vi "newOdometry.vi"(8 "Wheel angles":dbl[](array[numeric]), 9 "Wheel speed":dbl[](array[numeric]), 10 "prevSTR":dbl, 11 "prevFWD":dbl) -> (1 "Strafe":dbl, 2 "Forward":dbl)   [LabVIEW 2020]
uses:
  <vilib>/Rock Robotics/WPI/ThirdParty/Sensors/navX/_TypeDefs/FRIC_navX_DeviceNumbersTypeDef.ctl
  <vilib>/Rock Robotics/WPI/ThirdParty/JAS_Junk/TrajLib/Trajectory_Library.lvlib
panel:
  # "team 1684's odometry equation"
  # "0: Fl\n1: FR\n2: BL\n3: BR"
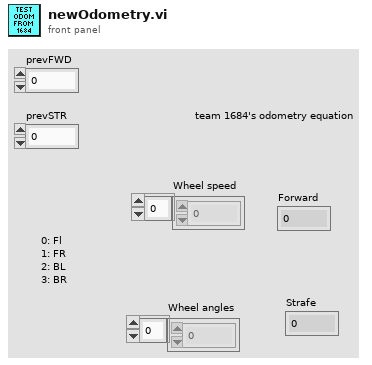
[diagram p1: front panel]
types:
  T1 = typedef "FRIC_navX_DeviceNumbersTypeDef.ctl" = enum16{"Dev0", "Dev1", "Dev2", "Dev3"}
  T2 = cluster{"Yaw":dbl, "Roll":dbl, "Pitch":dbl, "Heading":dbl, "Fused Heading":dbl}
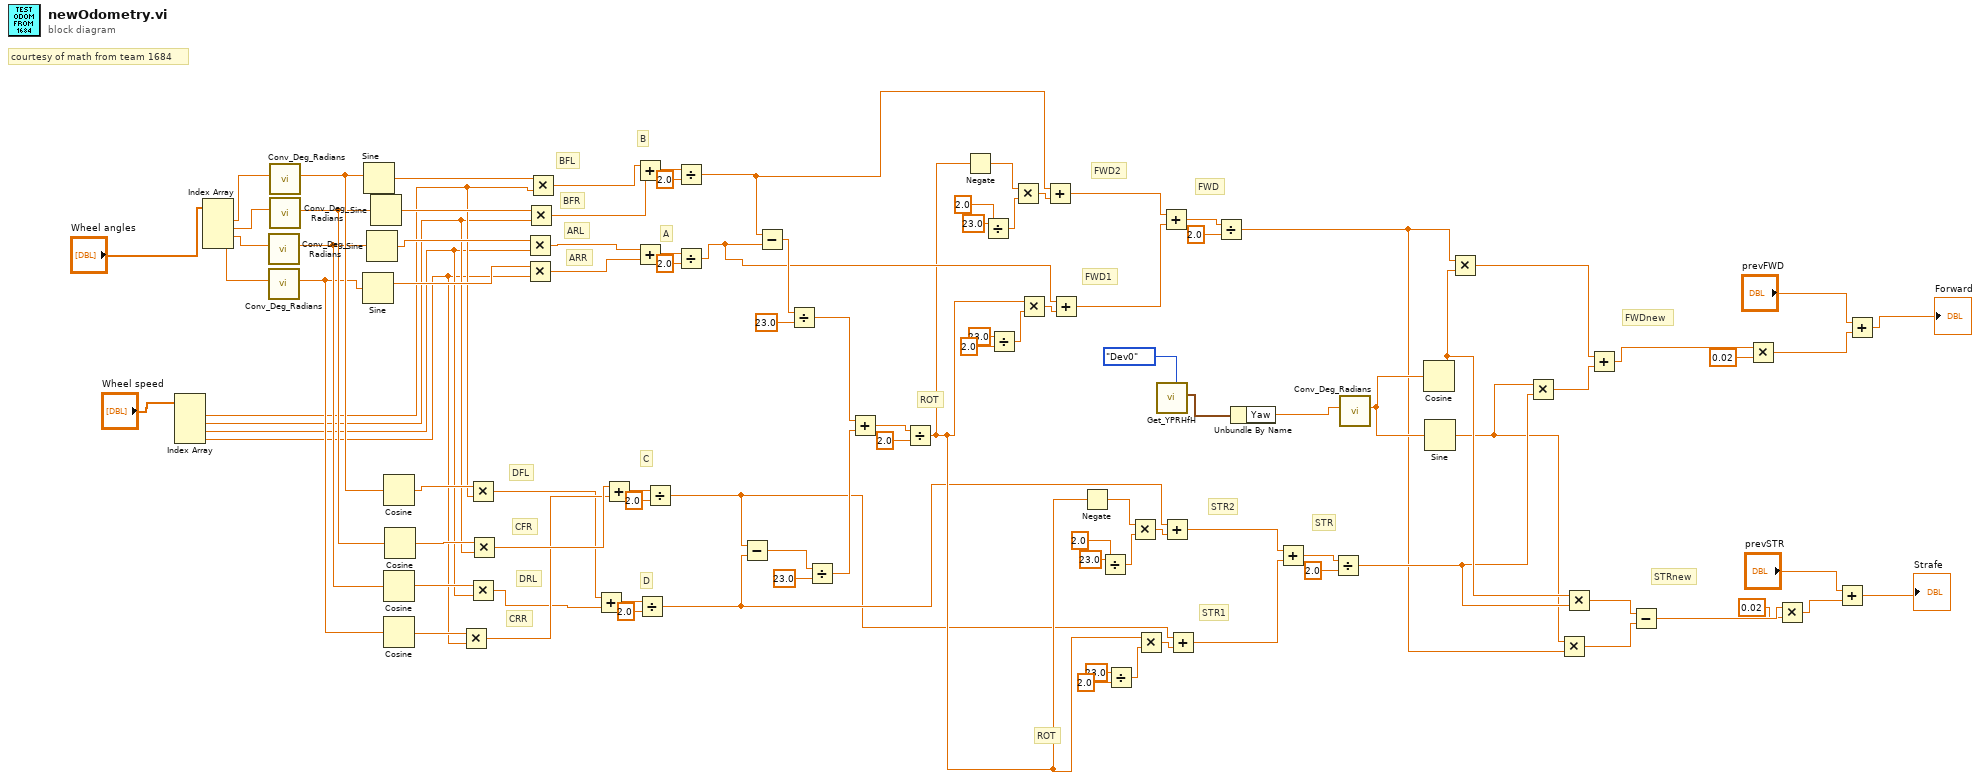
[diagram p0: block diagram]
diagram:
  # "STRnew"
  # "FWDnew"
  # "STR"
  # "STR2"
  # "STR1"
  # "ROT"
  # "FWD"
  # "FWD2"
  # "FWD1"
  # "ROT"
  # "D"
  # "C"
  # "A"
  # "B"
  # "CRR"
  # "DRL"
  # "CFR"
  # "DFL"
  # "ARR"
  # "ARL"
  # "BFR"
  # "BFL"
  # "courtesy of math from team 1684"
  n1 = Index Array(array="Wheel speed") -> (element #1=w83:dbl, element #2=w82:dbl, element #3=w81:dbl, element #4=w80:dbl)  [unwired: 4 in]
  n2 = Index Array(array="Wheel angles") -> (element #1=w99:dbl, element #2=w98:dbl, element #3=w97:dbl, element #4=w96:dbl)  [unwired: 4 in]
  n3 = call <vilib>:"Conv_Deg_Radians.vi"("Degress"=w97) -> ("Radians"=w89:dbl)  [unwired: 10 in]
  n4 = call <vilib>:"Conv_Deg_Radians.vi"("Degress"=w96) -> ("Radians"=w88:dbl)  [unwired: 10 in]
  n5 = call <vilib>:"Conv_Deg_Radians.vi"("Degress"=w99) -> ("Radians"=w91:dbl)  [unwired: 10 in]
  n6 = call <vilib>:"Conv_Deg_Radians.vi"("Degress"=w98) -> ("Radians"=w90:dbl)  [unwired: 10 in]
  n7 = Sine(x=w88) -> (sin(x)=w92:dbl)
  n8 = Sine(x=w91) -> (sin(x)=w95:dbl)
  n9 = Sine(x=w89) -> (sin(x)=w93:dbl)
  n10 = Sine(x=w90) -> (sin(x)=w94:dbl)
  n11 = Cosine(x=w91) -> (cos(x)=w87:dbl)
  n12 = Cosine(x=w89) -> (cos(x)=w85:dbl)
  n13 = Cosine(x=w88) -> (cos(x)=w84:dbl)
  n14 = Cosine(x=w90) -> (cos(x)=w86:dbl)
  n15 = Multiply(x=w84, y=w80) -> (x*y=w66:dbl)
  n16 = Multiply(x=w87, y=w83) -> (x*y=w65:dbl)
  n17 = Multiply(x=w85, y=w81) -> (x*y=w64:dbl)
  n18 = Multiply(x=w86, y=w82) -> (x*y=w67:dbl)
  n19 = Multiply(x=w93, y=w81) -> (x*y=w69:dbl)
  n20 = Multiply(x=w92, y=w80) -> (x*y=w68:dbl)
  n21 = Multiply(x=w94, y=w82) -> (x*y=w70:dbl)
  n22 = Multiply(x=w95, y=w83) -> (x*y=w71:dbl)
  n23 = Add(x=w65, y=w64) -> (x+y=w73:dbl)
  n24 = Add(x=w67, y=w66) -> (x+y=w75:dbl)
  n25 = Add(x=w71, y=w70) -> (x+y=w77:dbl)
  n26 = Add(x=w69, y=w68) -> (x+y=w79:dbl)
  n27 = Divide(x=w73, y=2.0) -> (x/y=w26:dbl)
  n28 = Divide(x=w75, y=2.0) -> (x/y=w25:dbl)
  n29 = Divide(x=w77, y=2.0) -> (x/y=w46:dbl)
  n30 = Divide(x=w79, y=2.0) -> (x/y=w51:dbl)
  n31 = Subtract(x=w25, y=w26) -> (x-y=w61:dbl)
  n32 = Subtract(x=w46, y=w51) -> (x-y=w62:dbl)
  n33 = Divide(x=w62, y=23.0) -> (x/y=w57:dbl)
  n34 = Divide(x=w61, y=23.0) -> (x/y=w56:dbl)
  n35 = Add(x=w57, y=w56) -> (x+y=w59:dbl)
  n36 = Divide(x=w59, y=2.0) -> (x/y=w29:dbl)
  n37 = Negate(x=w29) -> (-x=w47:dbl)
  n38 = Divide(x=23.0, y=2.0) -> (x/y=w50:dbl)
  n39 = Divide(x=23.0, y=2.0) -> (x/y=w54:dbl)
  n40 = Multiply(x=w47, y=w50) -> (x*y=w48:dbl)
  n41 = Multiply(x=w29, y=w54) -> (x*y=w52:dbl)
  n42 = Add(x=w46, y=w48) -> (x+y=w43:dbl)
  n43 = Add(x=w51, y=w52) -> (x+y=w42:dbl)
  n44 = Negate(x=w29) -> (-x=w34:dbl)
  n45 = Divide(x=23.0, y=2.0) -> (x/y=w37:dbl)
  n46 = Divide(x=23.0, y=2.0) -> (x/y=w40:dbl)
  n47 = Multiply(x=w34, y=w37) -> (x*y=w35:dbl)
  n48 = Multiply(x=w29, y=w40) -> (x*y=w38:dbl)
  n49 = call <vilib>:"Get_YPRHfH.vi"("Device Number"=FRIC_navX_DeviceNumbersTypeDef."Dev0") -> ("YRPHfH"=w23:T2)  [unwired: 10 in]
  n50 = Add(x=w43, y=w42) -> (x+y=w45:dbl)
  n51 = Add(x=w26, y=w35) -> (x+y=w31:dbl)
  n52 = Add(x=w25, y=w38) -> (x+y=w30:dbl)
  n53 = Divide(x=w45, y=2.0) -> (x/y=w15:dbl)
  n54 = Unbundle By Name(w23) -> ("Yaw"=w22:dbl)
  n55 = Add(x=w31, y=w30) -> (x+y=w33:dbl)
  n56 = Divide(x=w33, y=2.0) -> (x/y=w17:dbl)
  n57 = call <vilib>:"Conv_Deg_Radians.vi"("Degress"=w22) -> ("Radians"=w20:dbl)  [unwired: 10 in]
  n58 = Cosine(x=w20) -> (cos(x)=w18:dbl)
  n59 = Sine(x=w20) -> (sin(x)=w16:dbl)
  n60 = Multiply(x=w15, y=w18) -> (x*y=w21:dbl)
  n61 = Multiply(x=w16, y=w17) -> (x*y=w19:dbl)
  n62 = Multiply(x=w16, y=w15) -> (x*y=w13:dbl)
  n63 = Multiply(x=w18, y=w17) -> (x*y=w14:dbl)
  n64 = Add(x=w21, y=w19) -> (x+y=w11:dbl)
  n65 = Subtract(x=w14, y=w13) -> (x-y=w8:dbl)
  n66 = Multiply(x=w11, y=0.02) -> (x*y=w9:dbl)
  n67 = Multiply(x=w8, y=0.02) -> (x*y=w6:dbl)
  n68 = Add(x="prevSTR", y=w6) -> (x+y=→"Strafe":dbl)
  n69 = Add(x="prevFWD", y=w9) -> (x+y=→"Forward":dbl)
